vi "Periodic String Filter(variant).vi"(0 "Input String":string, 1 "reset?":bool, 2 "State":T1, 5 "Parameter":string, 9 "Remove Immediately?(F)":bool, 11 "Settings":T2={"threashold(#/s)"=1.0, "Check Peroid(s)"=1.0}) -> (4 "Input String(dup)":string, 8 ">> String-Parameter Map >>":variant=variant("CSM Tiny.DAQ: Break Continuous"=variant(u32 953145328), "CSM Tiny.DAQ: Close"=variant(u32 953145328), "CSM Tiny.DAQ: Configure"=variant(u32 953126122), "CSM Tiny.DAQ: Continuous Check"=variant(u32 953144928), "CSM Tiny.DAQ: Initialize"=variant(u32 953126122), "CSM Tiny.DAQ: Start"=variant(u32 953126122), "CSM Tiny.DAQ: Stop"=variant(u32 953145328), "CSM Tiny.Data"=variant(u32 953144928), "CSM Tiny.Data: Acquisite"=variant(u32 953144928), "CSM Tiny.UI: Refresh Buttons"=variant(u32 953145328)), 10 "Filtered Status":T3[](array[typedef]), 13 "added Info":string[](array[string]), 14 "removed info":T3[](array[typedef]), 15 "filtered?":bool)   [LabVIEW 2017, in "Communicable State Machine.lvlib"]
uses:
  user.lib/_NEVSTOP/Communicable State Machine(CSM)/Utility/Periodic String Filter Info.ctl
  user.lib/_NEVSTOP/Communicable State Machine(CSM)/Utility/Periodic String Filter State.ctl
  user.lib/_NEVSTOP/Communicable State Machine(CSM)/Communicable State Machine.lvlib
panel:
  out ">> Log Last Update Timestamp Map >>":variant=variant("CSM Tiny.DAQ: Break Continuous"=variant(u32 953145328), "CSM Tiny.DAQ: Close"=variant(u32 953145328), "CSM Tiny.DAQ: Configure"=variant(u32 953126122), "CSM Tiny.DAQ: Continuous Check"=variant(u32 953144928), "CSM Tiny.DAQ: Initialize"=variant(u32 953126122), "CSM Tiny.DAQ: Start"=variant(u32 953126122), "CSM Tiny.DAQ: Stop"=variant(u32 953145328), "CSM Tiny.Data"=variant(u32 953144928), "CSM Tiny.Data: Acquisite"=variant(u32 953144928), "CSM Tiny.UI: Refresh Buttons"=variant(u32 953145328))
  out ">> Log Count Map >>":variant=variant("CSM Tiny.DAQ: Break Continuous"=variant(i64 1), "CSM Tiny.DAQ: Close"=variant(i64 1), "CSM Tiny.DAQ: Configure"=variant(i64 1), "CSM Tiny.DAQ: Continuous Check"=variant(i64 192), "CSM Tiny.DAQ: Initialize"=variant(i64 1), "CSM Tiny.DAQ: Start"=variant(i64 1), "CSM Tiny.DAQ: Stop"=variant(i64 1), "CSM Tiny.Data"=variant(i64 97), "CSM Tiny.Data: Acquisite"=variant(i64 97), "CSM Tiny.UI: Refresh Buttons"=variant(i64 3))
  out ">> Log Last Check Count Map >>":variant=variant("CSM Tiny.DAQ: Break Continuous"=variant(i64 1), "CSM Tiny.DAQ: Close"=variant(i64 1), "CSM Tiny.DAQ: Configure"=variant(i64 1), "CSM Tiny.DAQ: Continuous Check"=variant(i64 188), "CSM Tiny.DAQ: Initialize"=variant(i64 1), "CSM Tiny.DAQ: Start"=variant(i64 1), "CSM Tiny.DAQ: Stop"=variant(i64 1), "CSM Tiny.Data"=variant(i64 95), "CSM Tiny.Data: Acquisite"=variant(i64 95), "CSM Tiny.UI: Refresh Buttons"=variant(i64 2))
  out ">> Log Last Check Timestamp Map >>":variant=variant("CSM Tiny.DAQ: Break Continuous"=variant(u32 953145328), "CSM Tiny.DAQ: Close"=variant(u32 953145328), "CSM Tiny.DAQ: Configure"=variant(u32 953126122), "CSM Tiny.DAQ: Continuous Check"=variant(u32 953144928), "CSM Tiny.DAQ: Initialize"=variant(u32 953126122), "CSM Tiny.DAQ: Start"=variant(u32 953126122), "CSM Tiny.DAQ: Stop"=variant(u32 953145328), "CSM Tiny.Data"=variant(u32 953144928), "CSM Tiny.Data: Acquisite"=variant(u32 953144928), "CSM Tiny.UI: Refresh Buttons"=variant(u32 953145328))
  out ">> Filtered Log Count Map >>":variant=variant("CSM Tiny.DAQ: Break Continuous"=variant(i64 1), "CSM Tiny.DAQ: Close"=variant(i64 1), "CSM Tiny.DAQ: Configure"=variant(i64 1), "CSM Tiny.DAQ: Continuous Check"=variant(i64 188), "CSM Tiny.DAQ: Initialize"=variant(i64 1), "CSM Tiny.DAQ: Start"=variant(i64 1), "CSM Tiny.DAQ: Stop"=variant(i64 1), "CSM Tiny.Data"=variant(i64 95), "CSM Tiny.Data: Acquisite"=variant(i64 95), "CSM Tiny.UI: Refresh Buttons"=variant(i64 2))
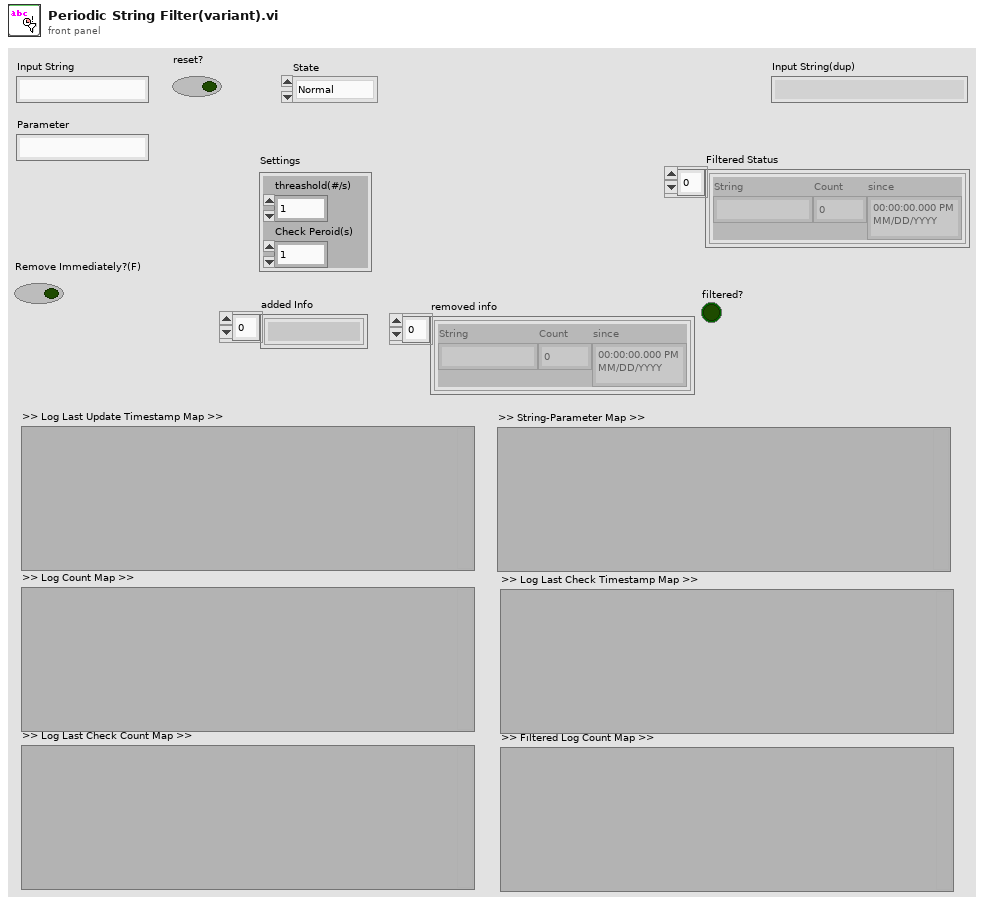
[diagram p1: front panel]
types:
  T1 = typedef "Communicable State Machine.lvlib/Periodic String Filter State.ctl" = enum16{"Normal", "Remove All Filters"}
  T2 = cluster{"threashold(#/s)":dbl, "Check Peroid(s)":dbl}
  T3 = typedef "Communicable State Machine.lvlib/Periodic String Filter Info.ctl" = cluster{"String":string, "Count":i64, "since":timestamp}
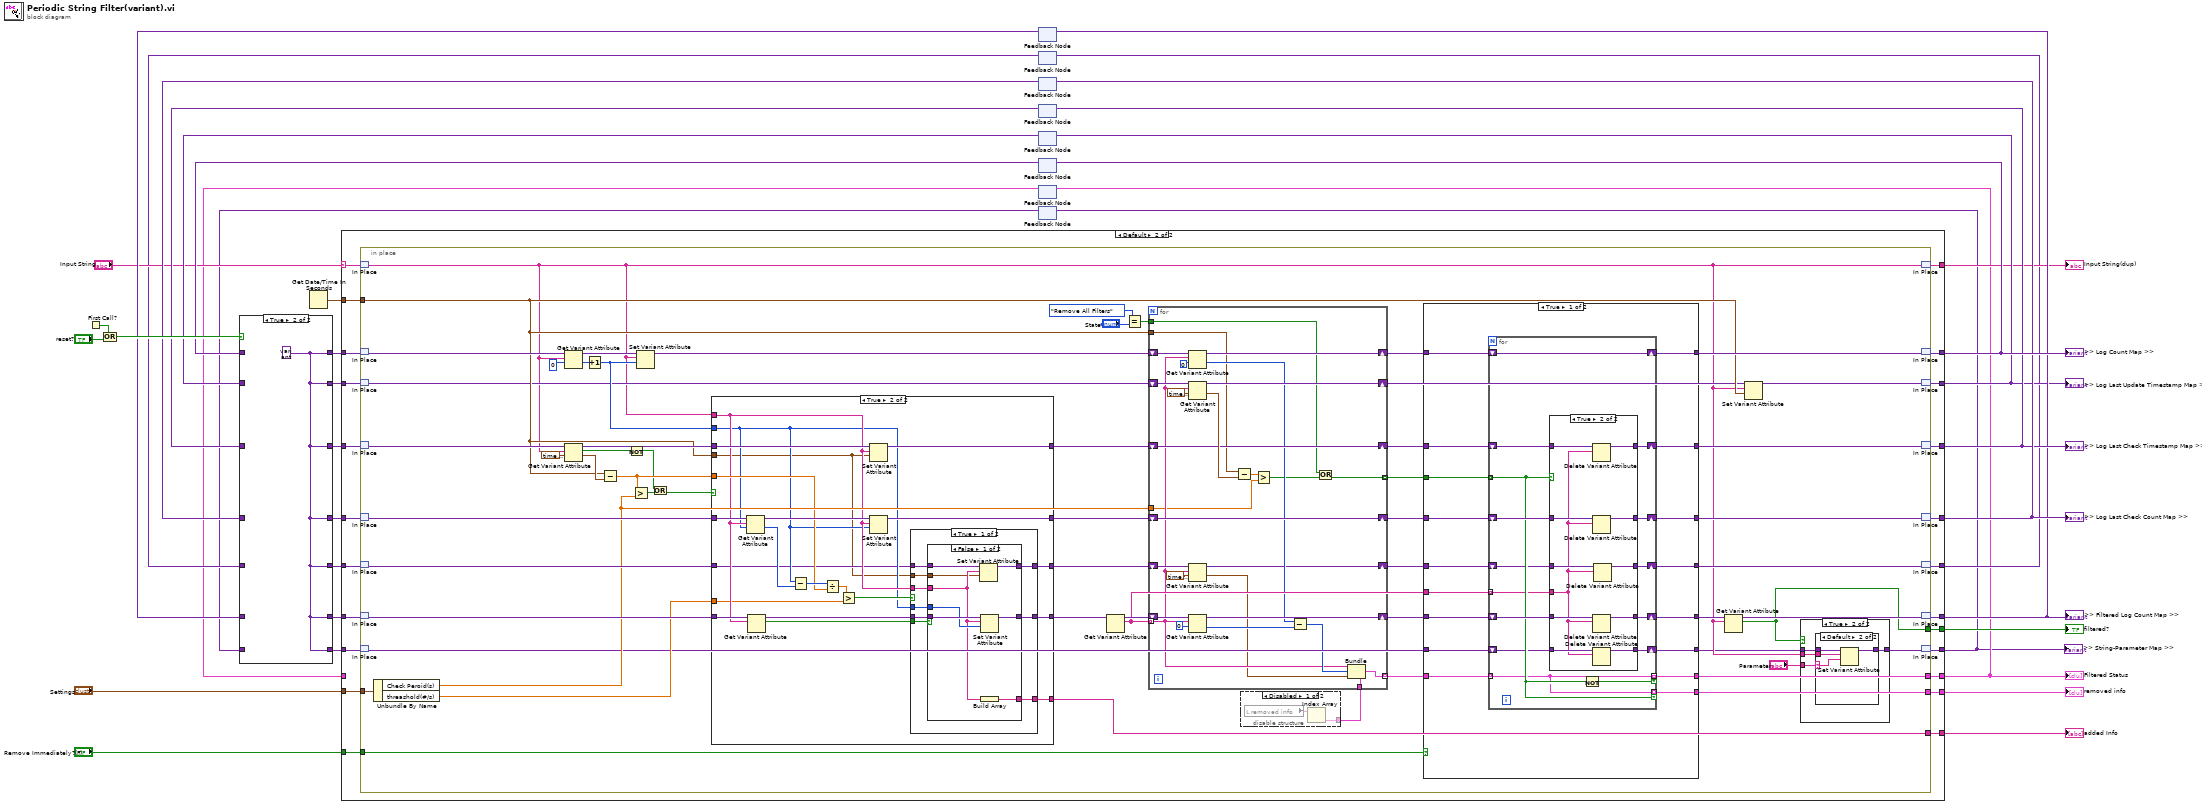
[diagram p0: block diagram]
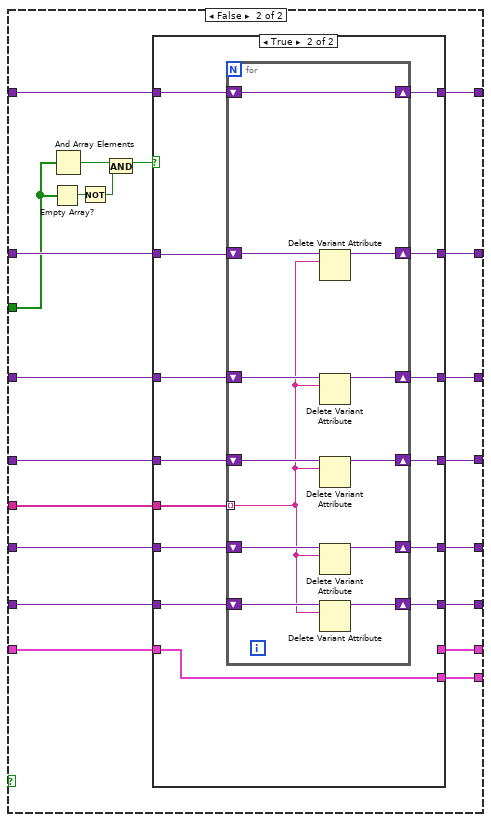
[diagram p6: hidden frame]
diagram:
  n1 = First Call?() -> (First Call?: T/F=w30:bool)
  n2 = Or(x=w30, y="reset?") -> (x .or. y?=w28:bool)
  n3 = Get Date/Time In Seconds() -> (seconds since 1Jan1904=w10:timestamp)
  n4 = feedback #1() -> (w24:variant)  [unwired: 1 in]
  n5 = feedback #2() -> (w8:variant)  [unwired: 1 in]
  n6 = feedback #3() -> (w21:variant)  [unwired: 1 in]
  n7 = feedback #4() -> (w23:variant)  [unwired: 1 in]
  n8 = feedback #5() -> (w18:variant)  [unwired: 1 in]
  n9 = feedback #6() -> (w26:variant)  [unwired: 1 in]
  n10 = feedback #7() -> (w5:T3[])  [unwired: 1 in]
  n11 = feedback #8() -> (w2:variant)  [unwired: 1 in]
  n12 = case shown="True" w28 {
    tunnel: [w41 w42] -> w27
    tunnel: w26 -> [w41 _]
    tunnel: [w40 w42] -> w25
    tunnel: w24 -> [w40 _]
    tunnel: w23 -> [w39 _]
    tunnel: [w39 w42] -> w22
    tunnel: w21 -> [w38 _]
    tunnel: [w38 w42] -> w20
    tunnel: [w37 w42] -> w19
    tunnel: w18 -> [w37 _]
    tunnel: [w36 w42] -> w9
    tunnel: w8 -> [w36 _]
    tunnel: [w35 w42] -> w3
    tunnel: w2 -> [w35 _]
    frame False {
    }
    frame True {
      w42 = variant
    }
  }
  n13 = case shown="Default" "Input String" {
    selector: "Input String" -> [_ w62]
    tunnel: [w50 w73] -> w34
    tunnel: [w47 w72] -> w33
    tunnel: [w48 w71] -> w32
    tunnel: [_ w70] -> w31
    tunnel: w27 -> [w50 w69]
    tunnel: w25 -> [w45 w68]
    tunnel: w22 -> [w48 w67]
    tunnel: w20 -> [w47 w66]
    tunnel: w19 -> [w49 w65]
    tunnel: [w45 w64] -> w17
    tunnel: [w49 w63] -> w16
    tunnel: [_ w61] -> w14
    tunnel: [w44 w60] -> w6
    tunnel: [_ w59] -> w13
    tunnel: [_ w58] -> w12
    tunnel: "Remove Immediately?(F)" -> [_ w57]
    tunnel: w10 -> [_ w56]
    tunnel: w9 -> [w46 w55]
    tunnel: [w46 w54] -> w7
    tunnel: w5 -> [w44 _]
    tunnel: "Settings" -> [_ w53]
    tunnel: w3 -> [w43 w52]
    tunnel: [w43 w51] -> w1
    frame "" {
    }
    frame Default {
      n14 = in-place {
        in-place-border: [w79] -> w70
        in-place-border: [w97] -> w60
        in-place-border: [w100] -> w59
        in-place-border: [w110] -> w58
        in-place-border: w57 -> [w103]
        in-place-border: w56 -> [w95]
        in-place-border: w53 -> [w90]
        n15 = in-place-match #9(w62) -> (w78:string)
        n16 = in-place-match #10(w69) -> (w128:variant)
        n17 = in-place-match #11(w65) -> (w88:variant)
        n18 = in-place-match #12(w67) -> (w126:variant)
        n19 = in-place-match #13(w66) -> (w124:variant)
        n20 = in-place-match #14(w55) -> (w94:variant)
        n21 = in-place-match #15(w68) -> (w122:variant)
        n22 = in-place-match #16(w52) -> (w77:variant)
        n23 = Unbundle By Name(w90) -> ("Check Peroid(s)"=w85:dbl, "threashold(#/s)"=w89:dbl)
        n24 = Get Variant Attribute(Variant=w128, name=w78, default value (empty Variant)=i64 0 ("64bit integer")) -> (duplicate Variant=w129:variant, value=w130:i64)  [unwired: 1 in, 2 out]
        n25 = Get Variant Attribute(Variant=w126, name=w78, default value (empty Variant)=timestamp(0 s since 1904-01-01) ("current time")) -> (duplicate Variant=w127:variant, found=w117:bool, value=w125:timestamp)  [unwired: 1 in, 1 out]
        n26 = Increment(x=w130) -> (x+1=w123:i64)
        n27 = Subtract(x=w95, y=w125) -> (x-y=w121:dbl)
        n28 = Not(x=w117) -> (.not. x?=w116:bool)
        n29 = Greater?(x=w121, y=w85) -> (0:w119:bool)
        n30 = Set Variant Attribute(Variant=w129, name=w78, value=w123) -> (Variant out=w112:variant)  [unwired: 1 in, 2 out]
        n31 = Or(x=w116, y=w119) -> (x .or. y?=w118:bool)
        n32 = case shown="True" w118 {
          tunnel: w127 -> [w277 w298]
          tunnel: [w277 w297] -> w114
          tunnel: w95 -> [_ w279]
          tunnel: w124 -> [w276 w295]
          tunnel: [w276 w296] -> w113
          tunnel: w123 -> [_ w283]
          tunnel: w78 -> [_ w285]
          tunnel: w122 -> [w275 w287]
          tunnel: [w275 w292] -> w80
          tunnel: w121 -> [_ w288]
          tunnel: [_ w282] -> w110
          tunnel: w94 -> [w274 w281]
          tunnel: [w274 w280] -> w93
          tunnel: w89 -> [_ w278]
          frame False {
          }
          frame True {
            n33 = Get Variant Attribute(Variant=w295, name=w285, default value (empty Variant)=w283) -> (duplicate Variant=w294:variant, value=w293:i64)  [unwired: 1 in, 2 out]
            n34 = Get Variant Attribute(Variant=w287, name=w285) -> (duplicate Variant=w286:variant, found=w284:bool)  [unwired: 2 in, 2 out]
            n35 = Subtract(x=w283, y=w293) -> (x-y=w290:i64)
            n36 = Divide(x=w290, y=w288) -> (x/y=w289:dbl)
            n37 = Greater?(x=w289, y=w278) -> (0:w291:bool)
            n38 = Set Variant Attribute(Variant=w298, name=w285, value=w279) -> (Variant out=w297:variant)  [unwired: 1 in, 2 out]
            n39 = Set Variant Attribute(Variant=w294, name=w285, value=w283) -> (Variant out=w296:variant)  [unwired: 1 in, 2 out]
            n40 = case shown="True" w291 {
              tunnel: w286 -> [w304 w319]
              tunnel: [w307 w319] -> w292
              tunnel: w285 -> [w305 _]
              tunnel: w283 -> [w306 _]
              tunnel: w284 -> [w303 _]
              tunnel: [w302 _] -> w282
              tunnel: w281 -> [w301 w318]
              tunnel: [w300 w318] -> w280
              tunnel: w279 -> [w299 _]
              frame True {
                n41 = case shown="False" w303 {
                  tunnel: [w314 w317] -> w307
                  tunnel: w304 -> [w315 w317]
                  tunnel: w305 -> [w309 _]
                  tunnel: w306 -> [w313 _]
                  tunnel: [w312 _] -> w302
                  tunnel: w301 -> [w311 w316]
                  tunnel: [w310 w316] -> w300
                  tunnel: w299 -> [w308 _]
                  frame False {
                    n42 = Set Variant Attribute(Variant=w311, name=w309, value=w308) -> (Variant out=w310:variant)  [unwired: 1 in, 2 out]
                    n43 = Set Variant Attribute(Variant=w315, name=w309, value=w313) -> (Variant out=w314:variant)  [unwired: 1 in, 2 out]
                    n44 = Build Array(w309) -> (w312:string[])
                  }
                  frame True {
                  }
                }
              }
              frame False {
              }
            }
          }
        }
        n45 = Get Variant Attribute(Variant=w80) -> (duplicate Variant=w115:variant, names=w98:string[])  [unwired: 3 in, 2 out]
        n46 = Equal?(x=Periodic_String_Filter_State."Remove All Filters", y="State") -> (x = y?=w81:bool)
        n47 = disable-structure shown="Disabled" {
          disable-tunnel: [w244 _] -> w84
          frame Disabled {
            n48 = local read "removed info"() -> (w245:T3[])
            n49 = Index Array(array=w245) -> (element=w244:T3)  [unwired: 1 in]
          }
          frame Enabled {
          }
        }
        n50 = for {
          tunnel: w98 -> [w252] mode=indexing
          shift-right: [w263] -> w104
          shift-left: w115 -> [w270]
          shift-right: [w271] -> w106
          shift-left: w113 -> [w271]
          shift-right: [w265] -> w108
          shift-left: w114 -> [w265]
          shift-right: [w266] -> w87
          shift-left: w88 -> [w267]
          shift-right: [w264] -> w102
          shift-left: w112 -> [w269]
          tunnel: [w257] -> w96 mode=indexing
          tunnel: [w247] -> w99 mode=indexing
          tunnel: w95 -> [w255]
          shift-right: [w250] -> w92
          shift-left: w93 -> [w254]
          tunnel: w85 -> [w249]
          tunnel: w84 -> [w248]
          tunnel: w81 -> [w246]
          n51 = Get Variant Attribute(Variant=w269, name=w252, default value (empty Variant)=i64 0) -> (duplicate Variant=w264:variant, value=w259:i64)  [unwired: 1 in, 2 out]
          n52 = Get Variant Attribute(Variant=w267, name=w252, default value (empty Variant)=timestamp(0 s since 1904-01-01) ("current time")) -> (duplicate Variant=w266:variant, value=w268:timestamp)  [unwired: 1 in, 2 out]
          n53 = Get Variant Attribute(Variant=w254, name=w252, default value (empty Variant)=timestamp(0 s since 1904-01-01) ("current time")) -> (duplicate Variant=w250:variant, value=w251:timestamp)  [unwired: 1 in, 2 out]
          n54 = Get Variant Attribute(Variant=w270, name=w252, default value (empty Variant)=i64 0) -> (duplicate Variant=w263:variant, value=w260:i64)  [unwired: 1 in, 2 out]
          n55 = Subtract(x=w255, y=w268) -> (x-y=w272:dbl)
          n56 = Greater?(x=w272, y=w249) -> (0:w256:bool)
          n57 = Subtract(x=w259, y=w260) -> (x-y=w258:i64)
          n58 = Or(x=w246, y=w256) -> (x .or. y?=w247:bool)
          n59 = Bundle(cluster=w248, "String"=w252, "Count"=w258, "since"=w251) -> (w257:T3)
        }
        n60 = case shown="True" w103 {
          tunnel: [w158 w210] -> w109
          tunnel: w108 -> [w157 w209]
          tunnel: [w156 w208] -> w107
          tunnel: w106 -> [w155 w207]
          tunnel: [w154 w206] -> w105
          tunnel: w104 -> [w150 w205]
          tunnel: w102 -> [w153 w200]
          tunnel: [w152 w199] -> w101
          tunnel: [w151 w198] -> w100
          tunnel: w99 -> [w148 w197]
          tunnel: w98 -> [w149 w196]
          tunnel: [w147 w195] -> w97
          tunnel: w96 -> [w144 w194]
          tunnel: w92 -> [w146 w193]
          tunnel: [w145 w192] -> w91
          tunnel: w77 -> [w142 w191]
          tunnel: [w143 w190] -> w76
          frame True {
            n61 = for {
              shift-right: [w172] -> w158
              shift-left: w157 -> [w173]
              shift-right: [w170] -> w156
              shift-left: w155 -> [w171]
              shift-right: [w169] -> w154
              shift-left: w150 -> [w167]
              tunnel: w149 -> [w162] mode=indexing
              shift-right: [w168] -> w152
              shift-left: w153 -> [w168]
              tunnel: [w161] -> w151 mode=indexing if=w166
              tunnel: w148 -> [w166] mode=indexing
              tunnel: [w161] -> w147 mode=indexing if=w165
              shift-right: [w164] -> w145
              shift-left: w146 -> [w163]
              tunnel: w144 -> [w161] mode=indexing
              shift-right: [w160] -> w143
              shift-left: w142 -> [w159]
              n62 = case shown="True" w166 {
                tunnel: w173 -> [w178 w189]
                tunnel: [w178 w188] -> w172
                tunnel: w171 -> [w177 w187]
                tunnel: [w177 w186] -> w170
                tunnel: [w176 w185] -> w169
                tunnel: w162 -> [_ w179]
                tunnel: w167 -> [w176 w184]
                tunnel: [w175 w183] -> w164
                tunnel: w163 -> [w175 w182]
                tunnel: [w174 w181] -> w160
                tunnel: w159 -> [w174 w180]
                frame False {
                }
                frame True {
                  n63 = Delete Variant Attribute(6:w179, 7:w189) -> (3:w188:variant)  [unwired: 1 in, 2 out]
                  n64 = Delete Variant Attribute(6:w179, 7:w187) -> (3:w186:variant)  [unwired: 1 in, 2 out]
                  n65 = Delete Variant Attribute(6:w179, 7:w184) -> (3:w185:variant)  [unwired: 1 in, 2 out]
                  n66 = Delete Variant Attribute(6:w179, 7:w180) -> (3:w181:variant)  [unwired: 1 in, 2 out]
                  n67 = Delete Variant Attribute(6:w179, 7:w182) -> (3:w183:variant)  [unwired: 1 in, 2 out]
                }
              }
              n68 = Not(x=w166) -> (.not. x?=w165:bool)
            }
          }
          frame False {
            n69 = Empty Array?(array=w197) -> (empty?=w202:bool)
            n70 = And Array Elements(Boolean array=w197) -> (logical AND=w203:bool)
            n71 = Not(x=w202) -> (.not. x?=w201:bool)
            n72 = And(x=w203, y=w201) -> (x .and. y?=w204:bool)
            n73 = case shown="True" w204 {
              tunnel: [w217 w230] -> w210
              tunnel: w209 -> [w217 w231]
              tunnel: [w216 w228] -> w208
              tunnel: w207 -> [w216 w229]
              tunnel: [w215 w227] -> w206
              tunnel: w205 -> [w215 w224]
              tunnel: w200 -> [w214 w226]
              tunnel: [w214 w225] -> w199
              tunnel: [_ w220] -> w198
              tunnel: w196 -> [_ w223]
              tunnel: [w213 _] -> w195
              tunnel: w194 -> [w213 w220]
              tunnel: w193 -> [w212 w222]
              tunnel: [w212 w221] -> w192
              tunnel: w191 -> [w211 w219]
              tunnel: [w211 w218] -> w190
              frame False {
              }
              frame True {
                n74 = for {
                  shift-right: [w242] -> w230
                  shift-left: w231 -> [w243]
                  shift-right: [w240] -> w228
                  shift-left: w229 -> [w241]
                  shift-right: [w239] -> w227
                  shift-left: w224 -> [w237]
                  tunnel: w223 -> [w232] mode=indexing
                  shift-right: [w238] -> w225
                  shift-left: w226 -> [w238]
                  shift-right: [w236] -> w221
                  shift-left: w222 -> [w235]
                  shift-right: [w233] -> w218
                  shift-left: w219 -> [w234]
                  n75 = Delete Variant Attribute(6:w232, 7:w243) -> (3:w242:variant)  [unwired: 1 in, 2 out]
                  n76 = Delete Variant Attribute(6:w232, 7:w241) -> (3:w240:variant)  [unwired: 1 in, 2 out]
                  n77 = Delete Variant Attribute(6:w232, 7:w235) -> (3:w236:variant)  [unwired: 1 in, 2 out]
                  n78 = Delete Variant Attribute(6:w232, 7:w237) -> (3:w239:variant)  [unwired: 1 in, 2 out]
                  n79 = Delete Variant Attribute(6:w232, 7:w234) -> (3:w233:variant)  [unwired: 1 in, 2 out]
                }
              }
            }
          }
        }
        n80 = Get Variant Attribute(Variant=w105, name=w78) -> (duplicate Variant=w120:variant, found=w79:bool)  [unwired: 2 in, 2 out]
        n81 = Set Variant Attribute(Variant=w87, name=w78, value=w95) -> (Variant out=w86:variant)  [unwired: 1 in, 2 out]
        n82 = case shown="True" w79 {
          tunnel: w76 -> [w132 w136]
          tunnel: w78 -> [_ w135]
          tunnel: [w132 w134] -> w75
          tunnel: "Parameter" -> [_ w133]
          frame False {
          }
          frame True {
            n83 = case shown="Default" w133 {
              selector: w133 -> [_ w138]
              tunnel: w136 -> [w137 w141]
              tunnel: w135 -> [_ w140]
              tunnel: [w137 w139] -> w134
              frame "" {
              }
              frame Default {
                n84 = Set Variant Attribute(Variant=w141, name=w140, value=w138) -> (Variant out=w139:variant)  [unwired: 1 in, 2 out]
              }
            }
          }
        }
        n85 = in-place-match #9(w78) -> (w61:string)
        n86 = in-place-match #10(w101) -> (w73:variant)
        n87 = in-place-match #11(w86) -> (w63:variant)
        n88 = in-place-match #12(w109) -> (w71:variant)
        n89 = in-place-match #13(w107) -> (w72:variant)
        n90 = in-place-match #14(w91) -> (w54:variant)
        n91 = in-place-match #15(w120) -> (w64:variant)
        n92 = in-place-match #16(w75) -> (w51:variant)
      }
    }
  }
  ">> Log Count Map >>" <- w34
  ">> Log Last Check Timestamp Map >>" <- w32
  ">> Log Last Check Count Map >>" <- w33
  "filtered?" <- w31
  ">> Filtered Log Count Map >>" <- w17
  ">> Log Last Update Timestamp Map >>" <- w16
  "Input String(dup)" <- w14
  "Filtered Status" <- w6
  "removed info" <- w13
  "added Info" <- w12
  ">> String-Parameter Map >>" <- w1
  n93 = feedback-in #1(w17) -> ()
  n94 = feedback-in #2(w7) -> ()
  n95 = feedback-in #3(w33) -> ()
  n96 = feedback-in #4(w32) -> ()
  n97 = feedback-in #5(w16) -> ()
  n98 = feedback-in #6(w34) -> ()
  n99 = feedback-in #7(w6) -> ()
  n100 = feedback-in #8(w1) -> ()
